vi "Week1_Slide47_DivideByZero.vi"() -> ()   [LabVIEW 2015]
panel:
  out "Error! Divide by zero!":bool
  out "x/y":dbl
  in  "y":dbl
  in  "stop":bool
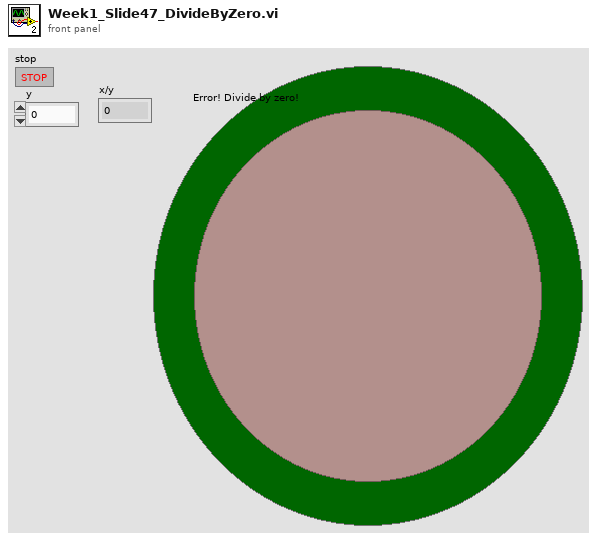
[diagram p1: front panel]
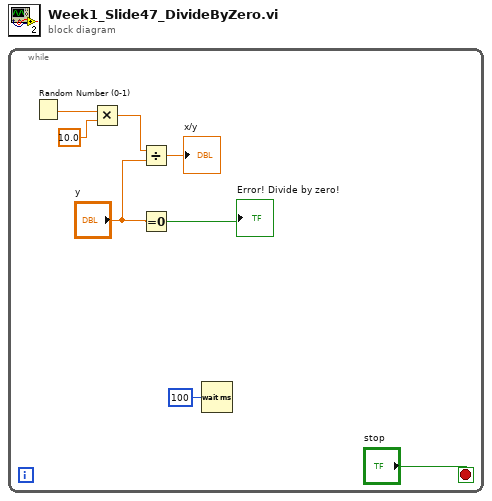
[diagram p0: block diagram]
diagram:
  n1 = while {
    stop <- "stop" stop-if-true
    n2 = Random Number (0-1)() -> (number: 0 to 1=w3:dbl)
    n3 = Multiply(x=w3, y=10.0) -> (x*y=w2:dbl)
    n4 = Divide(x=w2, y="y") -> (x/y=→"x/y":dbl)
    n5 = Equal To 0?(x="y") -> (x = 0?=→"Error! Divide by zero!":bool)
    n6 = Wait (ms)(milliseconds to wait=u32 100) -> ()  [unwired: 1 out]
  }
